vi "Class - ResultCntr.SectionEnd.vi"(8 "error in (no error)":errorcluster, 11 "Class - ResultCntr in":refnum<class "Class - ResultCntr.lvclass">) -> (0 "error out":errorcluster, 1 "ID":string, 3 "Class - ResultCntr out":refnum<class "Class - ResultCntr.lvclass">)   [LabVIEW 2017, in "Class - ResultCntr.lvclass"]
uses:
  Class - ResultCntr.lvclass
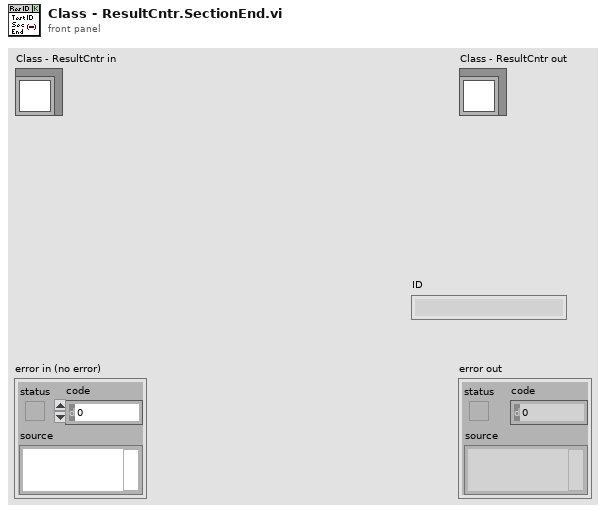
[diagram p1: front panel]
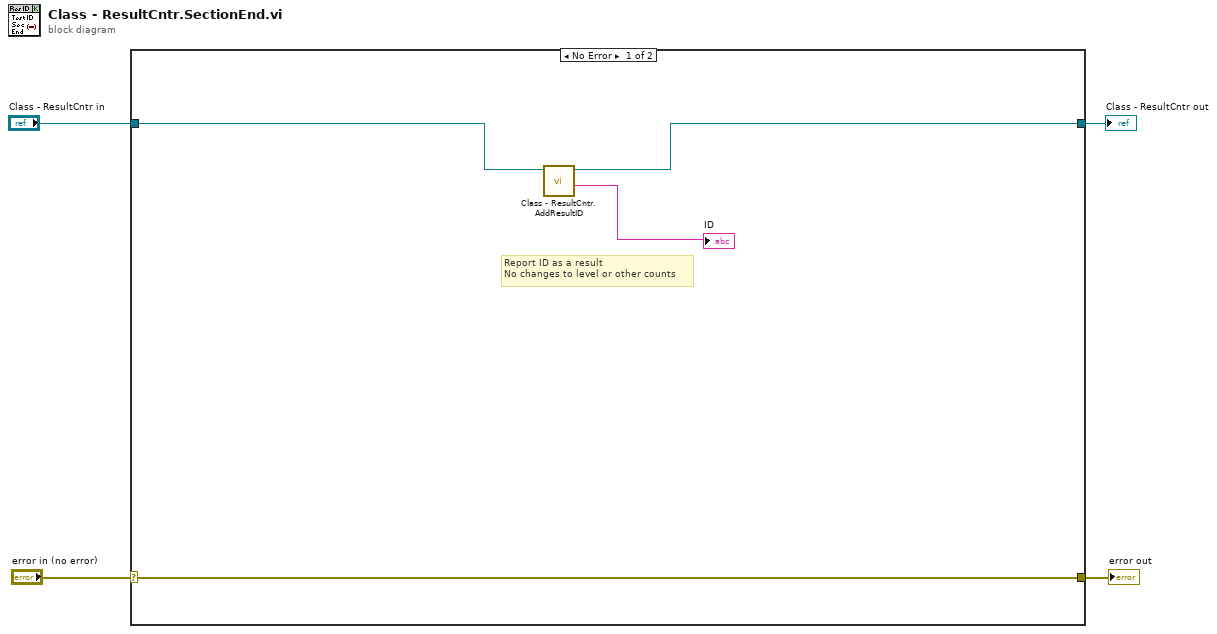
[diagram p0: block diagram]
diagram:
  n1 = case shown="No Error" "error in (no error)" {
    selector: "error in (no error)" -> [w8 w10]
    tunnel: [w8 w10] -> w3
    tunnel: [w6 w9] -> w1
    tunnel: "Class - ResultCntr in" -> [w7 w9]
    frame No Error {
      # "Report ID as a result\nNo changes to level or other counts"
      n2 = call "Class - ResultCntr.AddResultID.vi"("Class - ResultCntr in"=w7) -> ("ID"=→"ID":string, "Class - ResultCntr out"=w6:refnum<class "Class - ResultCntr.lvclass">)  [unwired: 8 in, 1 out]
    }
    frame Error {
    }
  }
  "error out" <- w3
  "Class - ResultCntr out" <- w1
